vi "GE 5565PIORC.DMA.Endianness.vi"(11 "count (1000)":u32=1000) -> (0 "error out":errorcluster, 3 "pass?":bool)   [LabVIEW 2017]
uses:
  Source/GE 5565PIORC.lvclass/GE 5565PIORC.ctl
  Source/Methods/GE 5565PIORC.DMA.Block.Write (DBL).vi
  Source/Methods/GE 5565PIORC.DMA.Create Transfer (Block).vi
  Source/Methods/GE 5565PIORC.DMA.Block.Read (DBL).vi
  Source/Properties/Registers/GE 5565PIORC.Registers.DMACSR0.Channel 0 Enable.Set.vi
  Source/Properties/GE 5565PIORC.Read VISA MEMACC.vi
  Source/Methods/GE 5565PIORC.DMA.Create Transfer (Scatter-Gather).vi
  Source/Methods/GE 5565PIORC.DMA.Configure.vi
  Source/Methods/GE 5565PIORC.PXI Interrupts.Discard Events.vi
  Source/Methods/GE 5565PIORC.DMA.Start.vi
  Source/Methods/GE 5565PIORC.DMA.Wait for Done.vi
  Source/Properties/Registers/GE 5565PIORC.Registers.Local Configuration.Read.vi
  Source/Properties/Registers/GE 5565PIORC.Registers.Local Configuration.Read (U8).vi
  Source/Properties/Registers/GE 5565PIORC.Registers.Local Configuration.Write.vi
  Source/Properties/Registers/GE 5565PIORC.Registers.Local Configuration.Write (U8).vi
  Source/Methods/GE 5565PIORC.Bit Manipulation.Set Bit.vi
  Source/Methods/GE 5565PIORC.Bit Manipulation.Set Bit (U8).vi
  Source/Methods/GE 5565PIORC.DMA.Size.vi
  Source/Properties/Registers/GE 5565PIORC.Registers.DMADPR0.Direction of Transfer.Set.vi
  Source/Properties/Registers/GE 5565PIORC.Registers.DMASIZ0.DMA Transfer Size.Set.vi
  Source/Properties/Registers/GE 5565PIORC.Registers.DMALADR0.Local Address Register.Set.vi
  Source/Properties/Registers/GE 5565PIORC.Registers.DMAMODE0.Scatter-Gather Mode.Set.vi
  Source/Properties/Registers/GE 5565PIORC.Registers.DMAPADR0.PCI Address Register.Set.vi
  Source/Methods/GE 5565PIORC.DMA.Scatter-Gather.Link Block Descriptors.vi
  Source/Methods/GE 5565PIORC.DMA.Scatter-Gather.Commit Linked Block Descriptors.vi
  Source/Properties/Registers/GE 5565PIORC.Registers.DMADPR0.Channel 0 First Descriptor Address.Set.vi
  Source/Methods/GE 5565PIORC.DMA.Get Transfer Components.vi
  Source/Methods/GE 5565PIORC.DMA.Get Transfer Components (Scatter-Gather).vi
  <vilib>/Utility/error.llb/Clear Errors.vi
  Source/Properties/Registers/GE 5565PIORC.Registers.DMACSR0.Channel 0 Start.Set.vi
  Source/Properties/Registers/GE 5565PIORC.Registers.DMACSR0.Channel 0 Clear Interrupt.Set.vi
  Source/Methods/GE 5565PIORC.DMA.Poll for Done Signal.vi
  Source/Methods/GE 5565PIORC.PXI Interrupts.Wait for Event.vi
  Source/Methods/GE 5565PIORC.Registers.Read.vi
  Source/Methods/GE 5565PIORC.Registers.Read (U8).vi
  Source/Methods/GE 5565PIORC.Registers.Write.vi
  Source/Methods/GE 5565PIORC.Registers.Write (U8).vi
  Source/Properties/Registers/GE 5565PIORC.Registers.Local Configuration.Read (U32).vi
  Source/Properties/Registers/GE 5565PIORC.Registers.Local Configuration.Write (U32).vi
  Source/Methods/GE 5565PIORC.Bit Manipulation.Set Bit (U32).vi
  Source/Methods/GE 5565PIORC.DMA.Scatter-Gather.Set Descriptor Params.vi
  Source/Methods/GE 5565PIORC.DMA.Is Done.vi
  Source/Methods/GE 5565PIORC.Registers.Read (U32).vi
  Source/Methods/GE 5565PIORC.Registers.Write (U32).vi
  Source/Properties/Registers/GE 5565PIORC.Registers.DMACSR0.Channel 0 Inactive.Get.vi
  Source/Methods/GE 5565PIORC.Bit Manipulation.Get Bit.vi
  Source/Methods/GE 5565PIORC.Bit Manipulation.Get Bit (U8).vi
  Source/Methods/GE 5565PIORC.Round Up to Nearest 8.vi
  Source/Methods/GE 5565PIORC.Round Up to Nearest 16.vi
  Source/GE 5565PIORC.lvclass
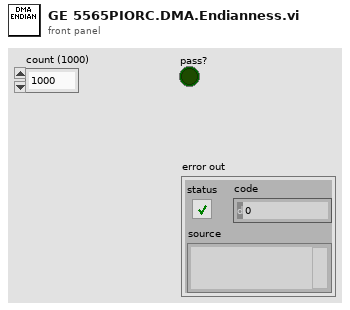
[diagram p1: front panel]
types:
  T1 = enum16{"big-endian, network order", "native, host order", "little-endian"}
  T2 = typedef "GE 5565PIORC.lvclass/GE 5565PIORC.Typedef.DMA Block Descriptor.ctl" = cluster{"descriptor ptr (VISA)":u32, "descriptor ptr (RFM)":u32, "descriptor size":u32, "descriptor params":T3}
  T3 = typedef "GE 5565PIORC.lvclass/GE 5565PIORC.Typedef.DMA Block Descriptor Params.ctl" = cluster{"data ptr (lower)":u32, "data ptr (upper)":u32, "data size":u32, "next descriptor ptr":u32}
  T4 = typedef "GE 5565PIORC.lvclass/GE 5565PIORC.Typedef.DMA Transfer Spec.ctl" = cluster{"RFM offset":u32, "Block Descriptors":T2[]}
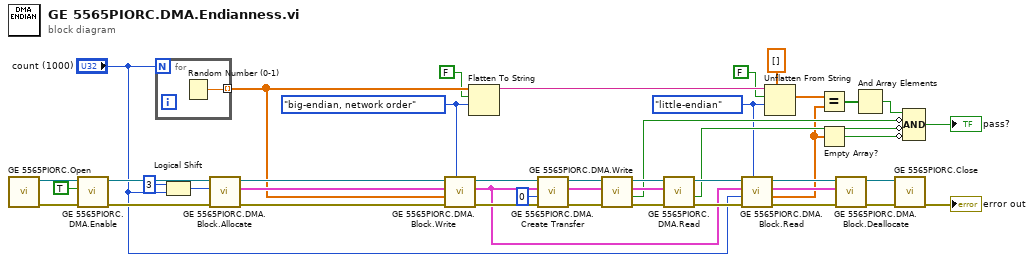
[diagram p0: block diagram]
diagram:
  w6 = T1."big-endian, network order" ("byte order (0:big-endian, network order)")
  w10 = T1."little-endian" ("byte order (0:big-endian, network order)")
  n1 = call "GE 5565PIORC.Open.vi"() -> ("error out"=w12:errorcluster, "GE 5565PIORC"=w13:refnum<class "GE 5565PIORC.lvclass">)  [unwired: 10 in]
  n2 = call "GE 5565PIORC.DMA.Enable.vi"("error in (no error)"=w12, "enable (T)"=TRUE ("Enable DMA"), "GE 5565PIORC in"=w13) -> ("error out"=w41:errorcluster, "GE 5565PIORC out"=w42:refnum<class "GE 5565PIORC.lvclass">)  [unwired: 7 in]
  n3 = for {
    N: "count (1000)" -> [_]
    tunnel: [w45] -> w5 mode=indexing
    n4 = Random Number (0-1)() -> (number: 0 to 1=w45:dbl)
  }
  n5 = Logical Shift(y=i16 3, x="count (1000)") -> (x << y=w36:u32)
  n6 = call "GE 5565PIORC.DMA.Block.Allocate.vi"("error in (no error)"=w41, "size in bytes"=w36, "GE 5565PIORC in"=w42) -> ("error out"=w38:errorcluster, "Block Descriptor"=w37:T2, "GE 5565PIORC out"=w39:refnum<class "GE 5565PIORC.lvclass">)  [unwired: 6 in]
  n7 = call-poly "GE 5565PIORC.DMA.Block.Write.vi"("byte order (big-endian)"=w6, "error in (no error)"=w38, "data"=w5, "Block Descriptor in"=w37, "GE 5565PIORC in"=w39) -> ("error out"=w33:errorcluster, "Block Descriptor out"=w30:T2, "GE 5565PIORC out"=w34:refnum<class "GE 5565PIORC.lvclass">)  [unwired: 3 in, 1 out]
  n8 = Flatten To String(anything=w5, prepend array or string size? (T)=FALSE, byte order (0:big-endian, network order)=w6) -> (data string=w11:string)  [unwired: 1 in, 2 out]
  n9 = call-poly "GE 5565PIORC.DMA.Create Transfer.vi"("error in (no error)"=w33, "RFM offset"=u32 0, "Block Descriptor"=w30, "GE 5565PIORC in"=w34) -> ("error out"=w19:errorcluster, "DMA Transfer Spec"=w18:T4, "GE 5565PIORC out"=w20:refnum<class "GE 5565PIORC.lvclass">)  [unwired: 4 in, 1 out]
  n10 = call "GE 5565PIORC.DMA.Write.vi"("error in (no error)"=w19, "DMA Transfer Spec"=w18, "GE 5565PIORC in"=w20) -> ("error out"=w15:errorcluster, "timed out?"=w14:bool, "DMA Transfer Spec dup"=w17:T4, "GE 5565PIORC out"=w16:refnum<class "GE 5565PIORC.lvclass">)  [unwired: 5 in]
  n11 = call "GE 5565PIORC.DMA.Read.vi"("error in (no error)"=w15, "DMA Transfer Spec"=w17, "GE 5565PIORC in"=w16) -> ("error out"=w31:errorcluster, "timed out?"=w26:bool, "GE 5565PIORC out"=w32:refnum<class "GE 5565PIORC.lvclass">)  [unwired: 5 in, 1 out]
  n12 = call-poly "GE 5565PIORC.DMA.Block.Read.vi"("byte order (big-endian)"=w10, "error in (no error)"=w31, "count"="count (1000)", "Block Descriptor in"=w30, "GE 5565PIORC in"=w32) -> ("error out"=w27:errorcluster, "data out"=w4:dbl[], "Block Descriptor out"=w28:T2, "GE 5565PIORC out"=w29:refnum<class "GE 5565PIORC.lvclass">)  [unwired: 3 in]
  n13 = Unflatten From String(type=dbl[] [] ("data out"), binary string=w11, data includes array or string size? (T)=FALSE, byte order (0:big-endian, network order)=w10) -> (value=w8:dbl[])  [unwired: 1 in, 2 out]
  n14 = Equal?(x=w8, y=w4) -> (x = y?=w25:bool[])
  n15 = Empty Array?(array=w4) -> (empty?=w3:bool)
  n16 = call "GE 5565PIORC.DMA.Block.Deallocate.vi"("error in (no error)"=w27, "Block Descriptor"=w28, "GE 5565PIORC in"=w29) -> ("error out"=w22:errorcluster, "GE 5565PIORC out"=w23:refnum<class "GE 5565PIORC.lvclass">)  [unwired: 7 in]
  n17 = And Array Elements(Boolean array=w25) -> (logical AND=w24:bool)
  n18 = call "GE 5565PIORC.Close.vi"("error in (no error)"=w22, "GE 5565PIORC"=w23) -> ("error out"=→"error out":errorcluster)  [unwired: 9 in]
  n19 = Compound Arithmetic op=AND(w24, invert w14, invert w26, invert w3) -> (→"pass?":bool)
